vi "SwerveDriveSystem.vi"(4 "Enable Auto Swerve Drive":bool, 5 "Automatic State Control Mode (F)":bool, 6 "Robot Motion Commands":T1, 7 "Robot field orientation (deg)":dbl, 8 "Drive Joystick Buttons":T4, 9 "Turn":dbl, 10 "Forward":dbl, 11 "Right":dbl) -> ()   [LabVIEW 2018]
uses:
  Controls/DriveJoystickButtonMapping.ctl
  Controls/Robot Pivot Motion Commands.ctl
  Controls/Pivot Motor Commands.ctl
  Controls/Robot Drive Mode.ctl
  Global Variables/reset gyro.vi
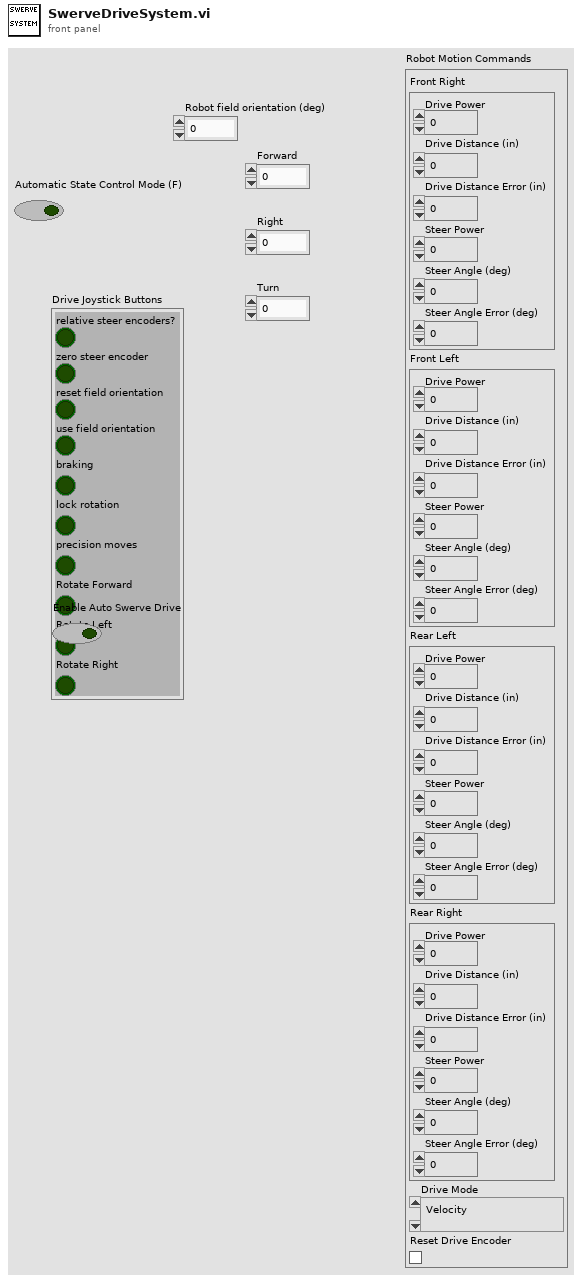
[diagram p1: front panel]
types:
  T1 = typedef "Robot Pivot Motion Commands.ctl" = cluster{"Front Right":T2, "Front Left":T2, "Rear Left":T2, "Rear Right":T2, "Drive Mode":T3, "Reset Drive Encoder":bool}
  T2 = typedef "Pivot Motor Commands.ctl" = cluster{"Drive Power":dbl, "Drive Distance (in)":dbl, "Drive Distance Error (in)":dbl, "Steer Power":dbl, "Steer Angle (deg)":dbl, "Steer Angle Error (deg)":dbl}
  T3 = typedef "Robot Drive Mode.ctl" = enum16{"Velocity", "Distance"}
  T4 = typedef "DriveJoystickButtonMapping.ctl" = cluster{"relative steer encoders?":bool, "zero steer encoder":bool, "reset field orientation":bool, "use field orientation":bool, "braking":bool, "lock rotation":bool, "precision moves":bool, "Rotate Forward":bool, "Rotate Left":bool, "Rotate Right":bool}
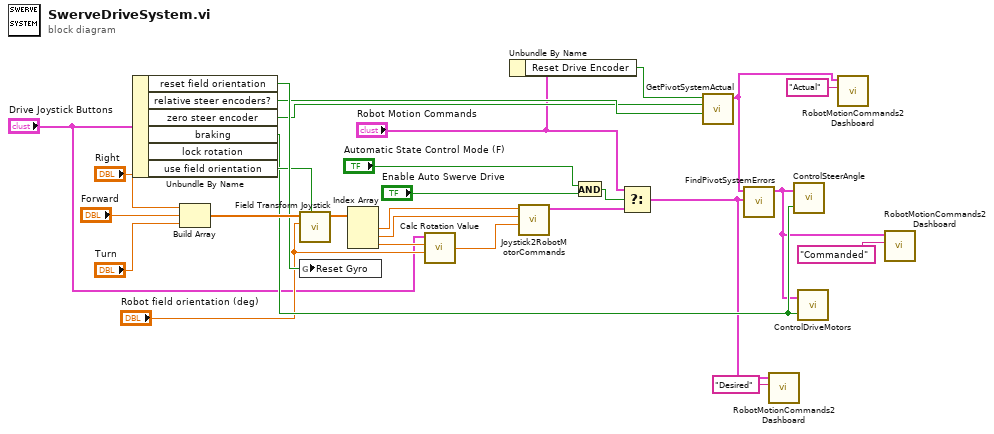
[diagram p0: block diagram]
diagram:
  n1 = Unbundle By Name("Drive Joystick Buttons") -> ("reset field orientation"=w22:bool, "relative steer encoders?"=w18:bool, "zero steer encoder"=w17:bool, "braking"=w16:bool, "use field orientation"=w20:bool)  [unwired: 1 out]
  n2 = Build Array("Right", "Forward", "Turn") -> (w23:dbl[])
  n3 = call "Field Transform Joystick.vi"("use field orientation"=w20, "robot field orientation (deg)"="Robot field orientation (deg)", "Joystick Values"=w23) -> ("Transformed Joystick Values"=w21:dbl[])  [unwired: 8 in]
  n4 = global write "reset gyro.vi" "Reset Gyro"(w22) -> ()
  n5 = Index Array(array=w21) -> (element #1=w28:dbl, element #2=w27:dbl, element #3=w4:dbl)  [unwired: 3 in]
  n6 = call "Calc Rotation Value.vi"("Gyro Angle"="Robot field orientation (deg)", "Joystick Rotation"=w4, "Rotation Data"="Drive Joystick Buttons") -> ("Rotation Value"=w2:dbl)  [unwired: 1 in]
  n7 = Unbundle By Name("Robot Motion Commands") -> ("Reset Drive Encoder"=w5:bool)
  n8 = call "Joystick2RobotMotorCommands.vi"("Joystick R"=w2, "Joystick Y"=w27, "Joystick X"=w28) -> ("Robot Motion Commands"=w19:T1)  [unwired: 8 in]
  n9 = And(x="Automatic State Control Mode (F)", y="Enable Auto Swerve Drive") -> (x .and. y?=w7:bool)
  n10 = Select(t="Robot Motion Commands", s=w7, f=w19) -> (s? t:f=w15:T1)
  n11 = call "GetPivotSystemActual.vi"("Relative Encoders?"=w18, "Zero Relative Encoder"=w17, "Zero Drive Encoder"=w5) -> ("Robot Motion Commands Out"=w12:T1)  [unwired: 8 in]
  n12 = call "FindPivotSystemErrors.vi"("Desired Motion"=w15, "Actual Pivot System"=w12) -> ("Commanded Motion"=w10:T1)  [unwired: 9 in]
  n13 = call "RobotMotionCommands2Dashboard.vi"("Label"="Desired", "Robot Motion Commands"=w15) -> ()  [unwired: 10 in]
  n14 = call "ControlSteerAngle.vi"("Braking"=w16, "Robot Motion Commands"=w10) -> ()  [unwired: 1 out]
  n15 = call "ControlDriveMotors.vi"("Braking"=w16, "Robot Motion Commands"=w10) -> ()  [unwired: 1 in]
  n16 = call "RobotMotionCommands2Dashboard.vi"("Label"="Actual", "Robot Motion Commands"=w12) -> ()  [unwired: 10 in]
  n17 = call "RobotMotionCommands2Dashboard.vi"("Label"="Commanded", "Robot Motion Commands"=w10) -> ()  [unwired: 10 in]
